vi "PWA_Fit.vi"(4 "polynomial order":i32=2, 5 "Input X^3":dbl[](array[numeric]) format="%.3f", 6 "Point selector":cluster{"Y":dbl, "X":dbl, "switch":bool}[](array[cluster]) {"X" format="%.2f"; "Y" format="%.2f"}, 7 "Input X^2":dbl[](array[numeric]) format="%.3f", 8 "Input X array":dbl[](array[numeric]) format="%.3f", 9 "Input Y array":dbl[](array[numeric]) format="%.4f") -> (0 "Point selector":cluster{"Y":dbl, "X":dbl, "switch":bool}[](array[cluster]) {"X" format="%.2f"; "Y" format="%.2f"}, 1 "Calibration plot":cluster{cluster{dbl, dbl}[]}[](graph), 2 "Coefficients":dbl[](array[numeric]) format="%.2f", 3 "Calib const":string[][](array[string]))   [LabVIEW 2010]
uses:
  Acquisition/PWA/PWAtasksGLOBAL.vi
panel:
  in  "Type":cluster{"Y":dbl, "X":dbl, "switch":bool}={"Y"=10.144154930121, "X"=9.20412, "switch"=FALSE} {"X" format="%.2f"; "Y" format="%.2f"}
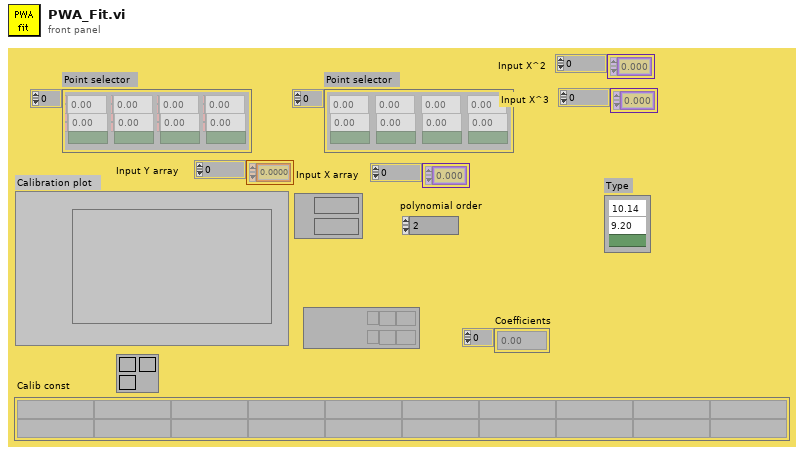
[diagram p1: front panel]
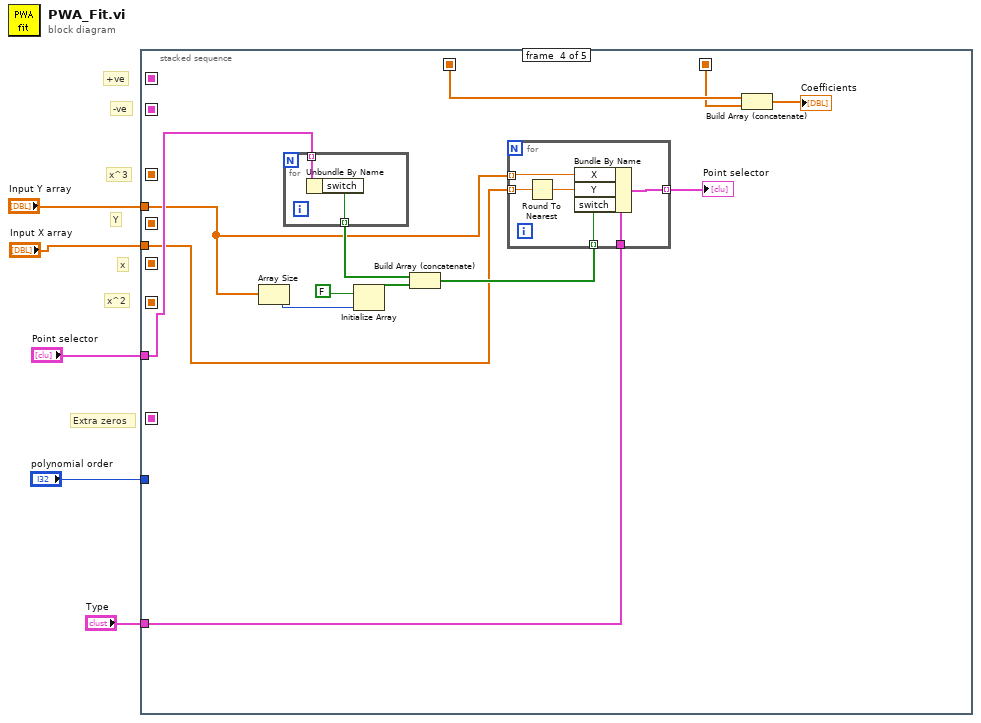
[diagram p0: block diagram]
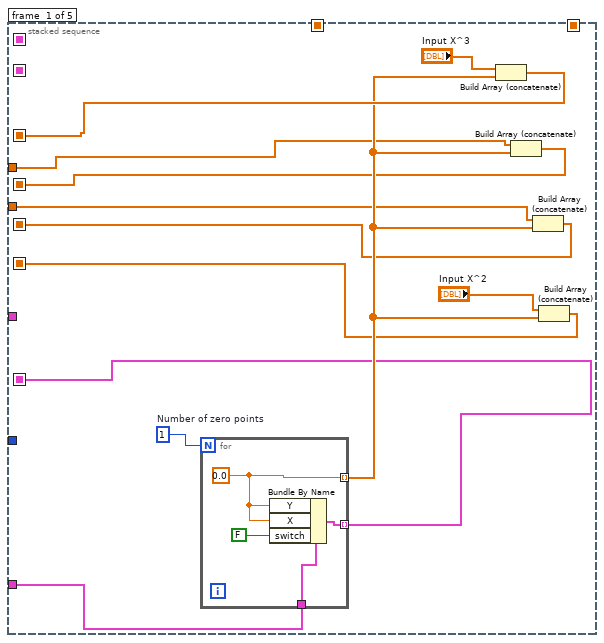
[diagram p2: hidden frame]
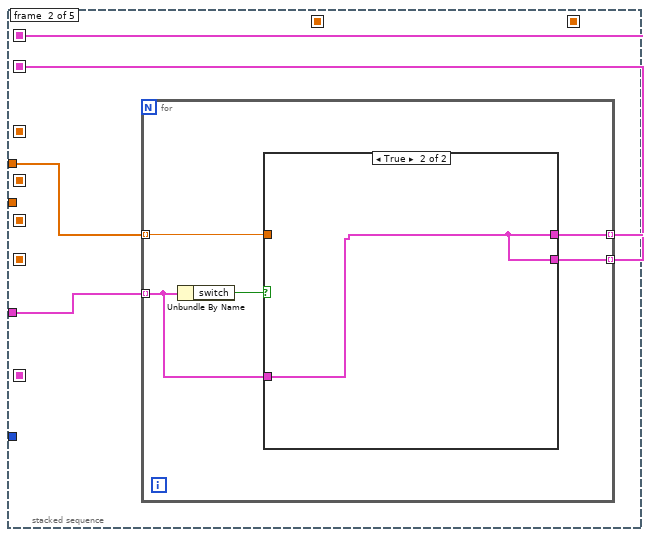
[diagram p3: hidden frame]
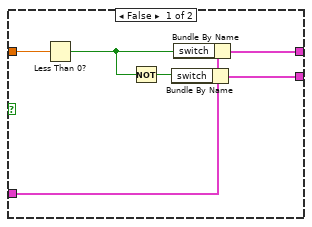
[diagram p4: hidden frame]
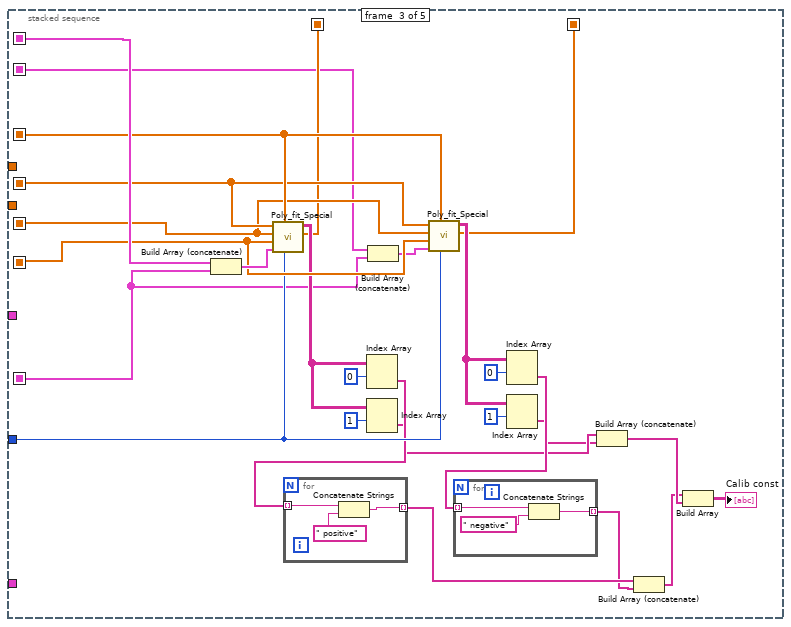
[diagram p5: hidden frame]
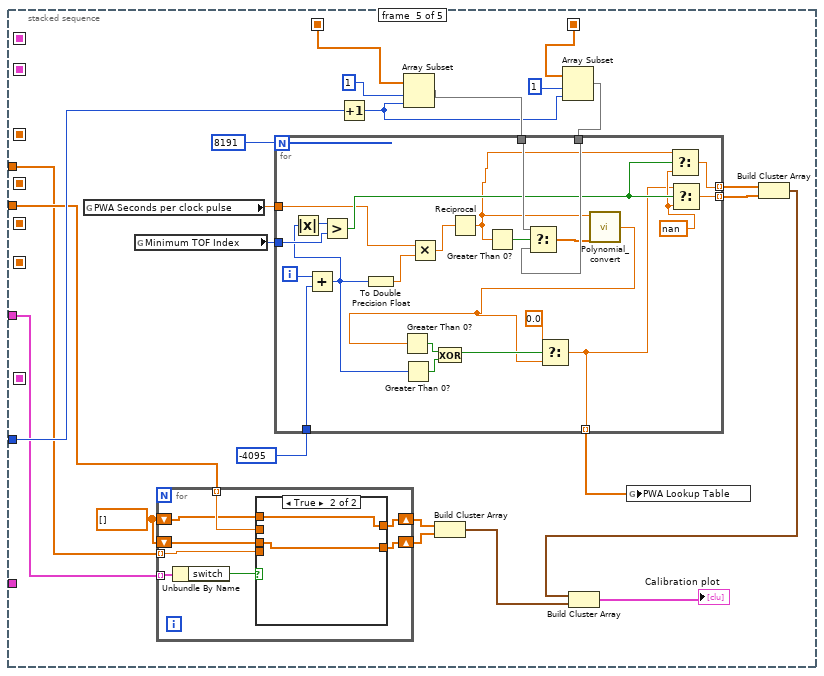
[diagram p6: hidden frame]
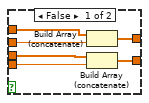
[diagram p7: hidden frame]
diagram:
  # "Extra zeros"
  # "Y"
  # "x^2"
  # "x"
  # "x^3"
  # "-ve"
  # "+ve"
  n1 = stacked-sequence {
    seq-local: [_ w25 _ _ _] -> [_ _ w64 _ _]
    seq-local: [_ w24 _ _ _] -> [_ _ w40 _ _]
    seq-local: [w14 _ _ _ _] -> [_ _ w62 _ _]
    seq-local: [w11 _ _ _ _] -> [_ _ w61 _ _]
    seq-local: [w10 _ _ _ _] -> [_ _ w60 _ _]
    seq-local: [w9 _ _ _ _] -> [_ _ w59 _ _]
    seq-local: [w7 _ _ _ _] -> [_ _ w39 _ _]
    seq-local: [_ _ w44 _ _] -> [_ _ _ w72 w111]
    seq-local: [_ _ w43 _ _] -> [_ _ _ w73 w113]
    tunnel: "Type" -> [w16 _ _ w75 _]
    tunnel: "Input Y array" -> [w8 w22 _ w77 w96]
    tunnel: "Point selector" -> [_ w23 _ w79 w98]
    tunnel: "Input X array" -> [w6 _ _ w76 w97]
    tunnel: "polynomial order" -> [_ _ w58 _ w114]
    frame #0 {
      w17 = 1  # Number of zero points
      n2 = for {
        N: w17 -> [_]
        tunnel: w16 -> [w21]
        tunnel: [w18] -> w12 mode=indexing
        tunnel: [w19] -> w7 mode=indexing
        w18 = 0.0
        n3 = Bundle By Name(cluster=w21, "Y"=w18, "X"=w18, "switch"=FALSE) -> (w19:cluster{"Y":dbl, "X":dbl, "switch":bool})
      }
      n4 = Build Array (concatenate)("Input X^3", w12) -> (w14:dbl[])
      n5 = Build Array (concatenate)(w8, w12) -> (w11:dbl[])
      n6 = Build Array (concatenate)(w6, w12) -> (w10:dbl[])
      n7 = Build Array (concatenate)("Input X^2", w12) -> (w9:dbl[])
    }
    frame #1 {
      n8 = for {
        tunnel: w23 -> [w28] mode=indexing
        tunnel: w22 -> [w29] mode=indexing
        tunnel: [w27] -> w25 mode=indexing
        tunnel: [w26] -> w24 mode=indexing
        n9 = Unbundle By Name(w28) -> ("switch"=w30:bool)
        n10 = case shown="True" w30 {
          tunnel: w29 -> [w36 _]
          tunnel: w28 -> [w35 w37]
          tunnel: [w32 w37] -> w27
          tunnel: [w31 w37] -> w26
          frame False {
            n11 = Less Than 0?(x=w36) -> (x < 0?=w33:bool)
            n12 = Not(x=w33) -> (.not. x?=w34:bool)
            n13 = Bundle By Name(cluster=w35, "switch"=w34) -> (w31:cluster{"Y":dbl, "X":dbl, "switch":bool})
            n14 = Bundle By Name(cluster=w35, "switch"=w33) -> (w32:cluster{"Y":dbl, "X":dbl, "switch":bool})
          }
          frame True {
          }
        }
      }
    }
    frame #2 {
      n15 = Build Array (concatenate)(w64, w39) -> (w63:cluster{"Y":dbl, "X":dbl, "switch":bool}[])
      n16 = call "Poly_fit_Special.vi"("polynomial order"=w58, "Input X^3"=w62, "Point selector"=w63, "Input X^2"=w59, "Input X array"=w60, "Input Y array"=w61) -> ("Coefficients"=w43:dbl[], "Calib const"=w55:string[][])  [unwired: 2 out]
      n17 = Index Array(array=w55, index (row)=0) -> (element=w51:string[])  [unwired: 1 in]
      n18 = for {
        tunnel: w51 -> [w70] mode=indexing
        tunnel: [w68] -> w49 mode=indexing
        n19 = Concatenate Strings(w70, " positive" ("string")) -> (w68:string)
      }
      n20 = Index Array(array=w55, index (row)=1) -> (element=w47:string[])  [unwired: 1 in]
      n21 = Build Array (concatenate)(w40, w39) -> (w38:cluster{"Y":dbl, "X":dbl, "switch":bool}[])
      n22 = call "Poly_fit_Special.vi"("polynomial order"=w58, "Input X^3"=w62, "Point selector"=w38, "Input X^2"=w59, "Input X array"=w60, "Input Y array"=w61) -> ("Coefficients"=w44:dbl[], "Calib const"=w52:string[][])  [unwired: 2 out]
      n23 = Index Array(array=w52, index (row)=0) -> (element=w50:string[])  [unwired: 1 in]
      n24 = for {
        tunnel: w50 -> [w67] mode=indexing
        tunnel: [w65] -> w48 mode=indexing
        n25 = Concatenate Strings(w67, " negative" ("string")) -> (w65:string)
      }
      n26 = Index Array(array=w52, index (row)=1) -> (element=w46:string[])  [unwired: 1 in]
      n27 = Build Array (concatenate)(w47, w46) -> (w42:string[])
      n28 = Build Array (concatenate)(w49, w48) -> (w41:string[])
      n29 = Build Array(w41, w42) -> (→"Calib const":string[][])
    }
    frame #3 {
      n30 = Array Size(array=w77) -> (size(s)=w82:i32)
      n31 = for {
        tunnel: w79 -> [w91] mode=indexing
        tunnel: [w90] -> w80 mode=indexing
        n32 = Unbundle By Name(w91) -> ("switch"=w90:bool)
      }
      n33 = Initialize Array(FALSE, w82) -> (w83:bool[])
      n34 = Build Array (concatenate)(w80, w83) -> (w78:bool[])
      n35 = for {
        tunnel: w77 -> [w84] mode=indexing
        tunnel: w76 -> [w86] mode=indexing
        tunnel: w78 -> [w89] mode=indexing
        tunnel: [w88] -> w74 mode=indexing
        tunnel: w75 -> [w87]
        n36 = Round To Nearest(number=w86) -> (nearest integer value=w85:dbl)
        n37 = Bundle By Name(cluster=w87, "X"=w84, "Y"=w85, "switch"=w89) -> (w88:cluster{"Y":dbl, "X":dbl, "switch":bool})
      }
      "Point selector" <- w74
      n38 = Build Array (concatenate)(w73, w72) -> (→"Coefficients":dbl[])
    }
    frame #4 {
      w93 = dbl[] []
      n39 = global read "PWAtasksGLOBAL.vi" "PWA Seconds per clock pulse"() -> (w92:dbl)
      n40 = global read "PWAtasksGLOBAL.vi" "Minimum TOF Index"() -> (w103:i16)
      n41 = for {
        tunnel: w98 -> [w123] mode=indexing
        shift-right: [w121] -> w95
        shift-left: w93 -> [w118]
        shift-right: [w122] -> w94
        shift-left: w93 -> [w117]
        tunnel: w97 -> [w120] mode=indexing
        tunnel: w96 -> [w119] mode=indexing
        n42 = Unbundle By Name(w123) -> ("switch"=w116:bool)
        n43 = case shown="True" w116 {
          tunnel: [w129 w130] -> w122
          tunnel: [w128 w131] -> w121
          tunnel: w120 -> [w127 _]
          tunnel: w119 -> [w126 _]
          tunnel: w118 -> [w125 w131]
          tunnel: w117 -> [w124 w130]
          frame False {
            n44 = Build Array (concatenate)(w125, w127) -> (w128:dbl[])
            n45 = Build Array (concatenate)(w124, w126) -> (w129:dbl[])
          }
          frame True {
          }
        }
      }
      n46 = Increment(x=w114) -> (x+1=w110:i32)
      n47 = Array Subset(array=w113, index=1, length=w110) -> (w112:dbl[])
      n48 = Build Cluster Array(w95, w94) -> (w115:cluster{dbl, dbl}[])
      n49 = Array Subset(array=w111, index=1, length=w110) -> (w109:dbl[])
      n50 = for {
        N: 8191 -> [_]
        tunnel: w112 -> [w154]
        tunnel: w109 -> [w153]
        tunnel: -4095 ("y") -> [w151]
        tunnel: w103 -> [w150]
        tunnel: [w145] -> w101 mode=indexing
        tunnel: [w146] -> w100 mode=indexing
        tunnel: [w135] -> w99 mode=indexing
        tunnel: w92 -> [w132]
        i -> [w152]
        w142 = nan
        n51 = Add(x=w152, y=w151) -> (x+y=w141:i32)
        n52 = Absolute Value(x=w141) -> (abs(x)=w149:i32)
        n53 = Greater?(x=w149, y=w150) -> (0:w144:bool)
        n54 = To Double Precision Float(number=w141) -> (double precision float=w134:dbl)
        n55 = Greater Than 0?(x=w141) -> (x > 0?=w139:bool)
        n56 = Multiply(x=w132, y=w134) -> (x*y=w133:dbl)
        n57 = Reciprocal(x=w133) -> (1/x=w143:dbl)
        n58 = Greater Than 0?(x=w143) -> (x > 0?=w148:bool)
        n59 = Select(t=w154, s=w148, f=w153) -> (s? t:f=w147:dbl[])
        n60 = call "Polynomial_convert.vi"("Calib constants"=w147, "Voltage"=w143) -> ("Eng Values"=w137:dbl)  [unwired: 4 out]
        n61 = Greater Than 0?(x=w137) -> (x > 0?=w140:bool)
        n62 = Exclusive Or(1:w139, 2:w140) -> (0:w138:bool)
        n63 = Select(t=0.0, s=w138, f=w137) -> (s? t:f=w135:dbl)
        n64 = Select(t=w143, s=w144, f=w142) -> (s? t:f=w145:dbl)
        n65 = Select(t=w135, s=w144, f=w142) -> (s? t:f=w146:dbl)
      }
      n66 = global write "PWAtasksGLOBAL.vi" "PWA Lookup Table"(w99) -> ()
      n67 = Build Cluster Array(w101, w100) -> (w102:cluster{dbl, "Eng Values":dbl}[])
      n68 = Build Cluster Array(w102, w115) -> (→"Calibration plot":cluster{cluster{dbl, "Eng Values":dbl}[]}[])
    }
  }
